vi "Process.vi"(8 "error in (no error)":errorcluster, 11 "SMO.UI.Example":refnum<class "SMO.UI.Example.lvclass">) -> (0 "error out":errorcluster, 3 "SMO.UI.Example out":refnum<class "SMO.UI.Example.lvclass">)   [LabVIEW 2013, in "SMO.UI.Example.lvclass"]
uses:
  SMO.UI.Example.lvclass
  src/SMO/Typedefs/Parent Call--Enum.ctl
  SMO.UI.Example.lvclass/SMO.UI.Example.ctl
  src/SMO.UI/SMO.UI.lvclass
  <vilib>/Utility/miscctls.llb/LVPointTypeDef.ctl
  SMO.Example/SMO.Example.lvclass
  src/SMO/SMO.lvclass
panel:
  in  "------------ User Events -------":bool=TRUE
  out "Waveform Chart":cluster{"Flow 2":dbl, "Flow 1":dbl}(graph)
  out "Sensor 1 (LPM)":u8
  out "Sensor 2 (LPM)":u8
  in  "Valve":bool
  in  "Pump":bool
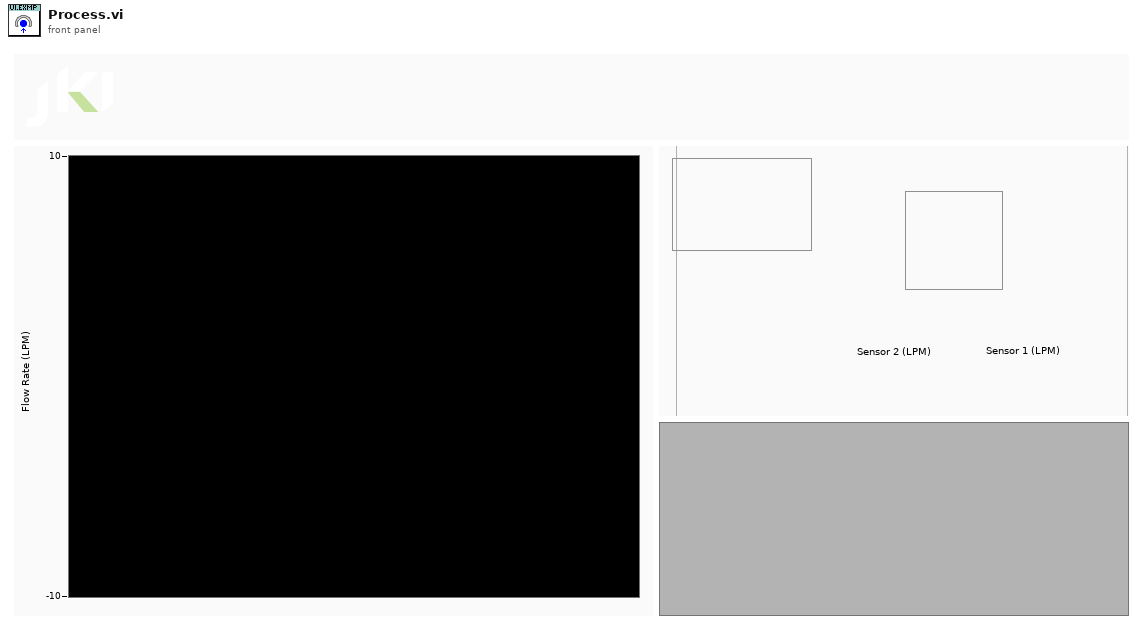
[diagram p1: front panel]
types:
  T1 = typedef "SMO.lvclass/Parent Call--Enum.ctl" = enum16{"Allows parent to run", "Does not request parent to run"}
  T2 = enum32{"invalid app kind", "Development System", "Run Time System", "Student Edition", "Embedded LabVIEW", "Evaluation", "Custom"}
  T3 = typedef "LVPointTypeDef.ctl" = cluster{"Horizontal":i16, "Vertical":i16}
  T4 = enum32{"Invalid", "Standard", "Closed", "Hidden", "Minimized", "Maximized"}
  T5 = typedef "SMO.UI.Example.lvclass/Dependencies--Cluster.ctl" = cluster{"SMO.Example":refnum<class "SMO.Example.lvclass">}
  T6 = cluster{"Core":cluster{"Current VI Reference":refnum<vi>, "Close Panel on Exit?":bool, "error":errorcluster}, "Self Ref":refnum<class "SMO.UI.Example.lvclass">, "Dependencies":T5, "Flow 1":dbl, "Flow 2":dbl, "Pump State":bool}
  T7 = cluster{"Current VI Reference":refnum<vi>, "Close Panel on Exit?":bool, "error":errorcluster}
  T8 = typedef "SMO.lvclass/Protected Events.ctl" = cluster{"StopProcesses":refnum<user-event>, "AbortProcesses":refnum<user-event>, "Config Changed":refnum<user-event>, "Dependency":refnum<user-event>}
  T9 = cluster{"Event Registration Refnum":refnum<event-registration>, "SMO.Example Public Events":refnum<event-registration>}
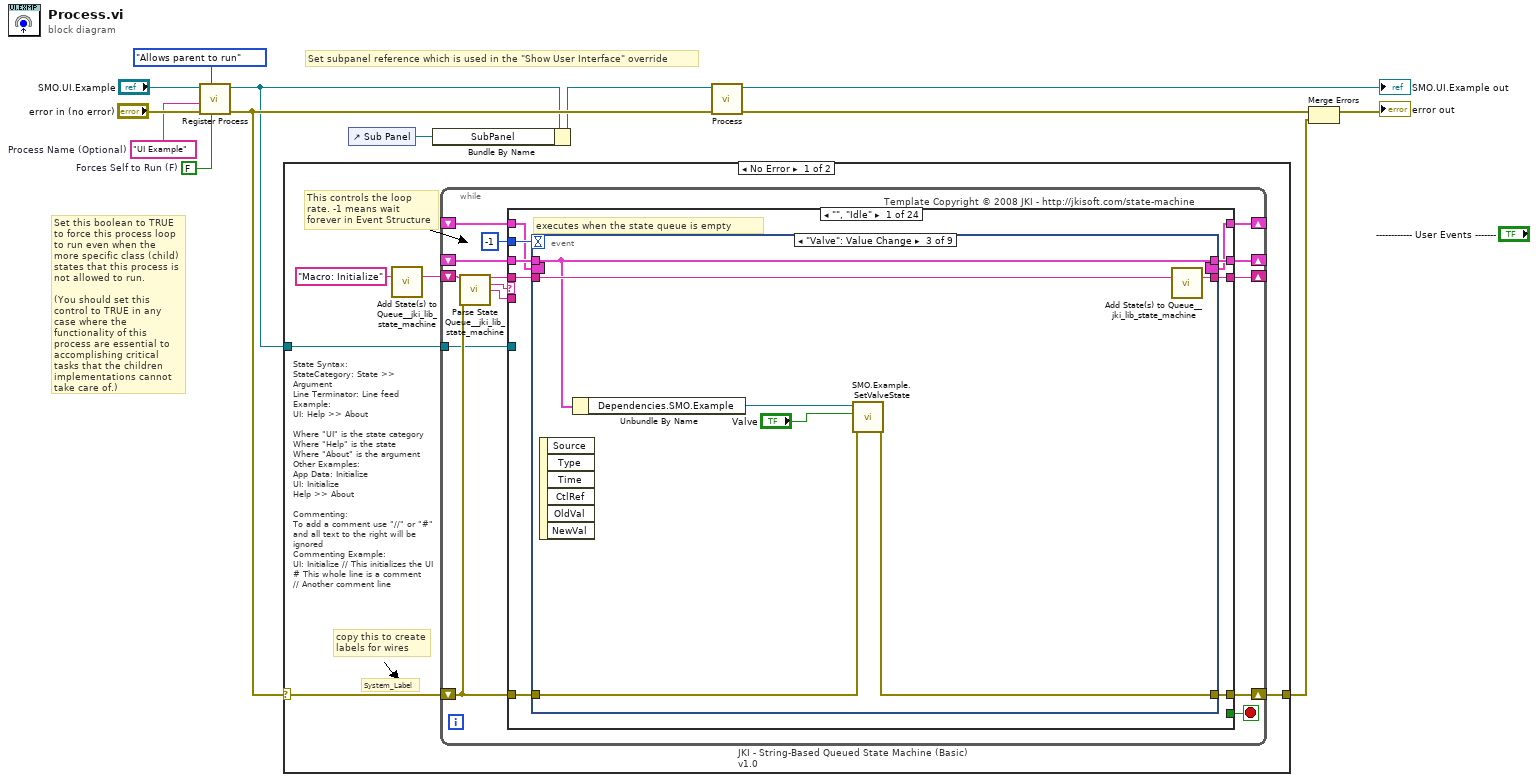
[diagram p0: block diagram]
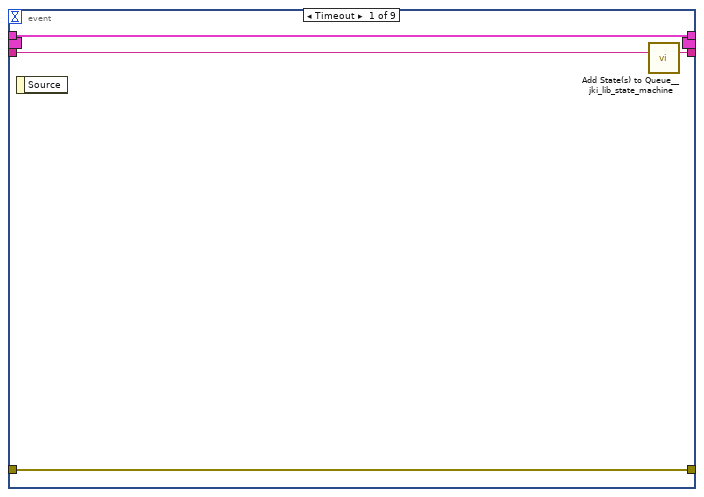
[diagram p2: hidden frame]
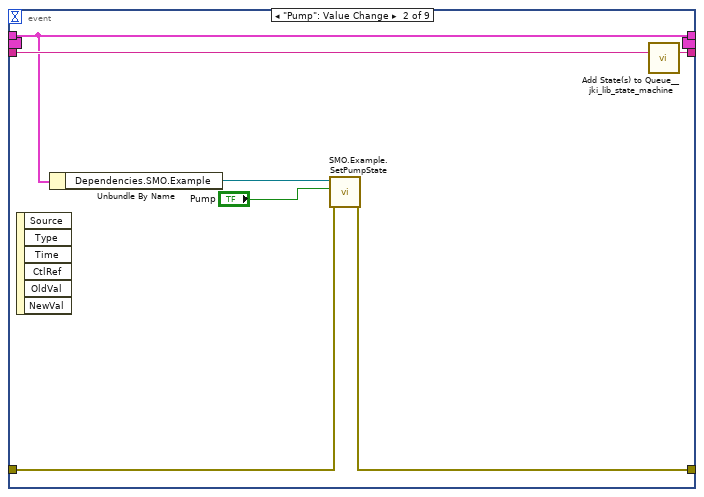
[diagram p3: hidden frame]
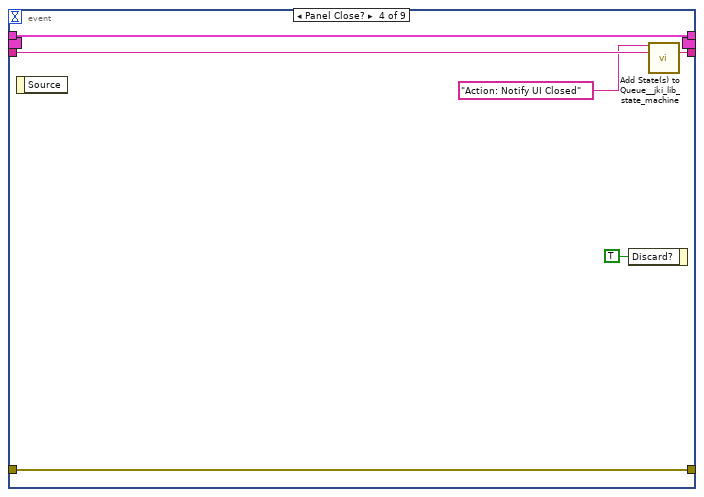
[diagram p4: hidden frame]
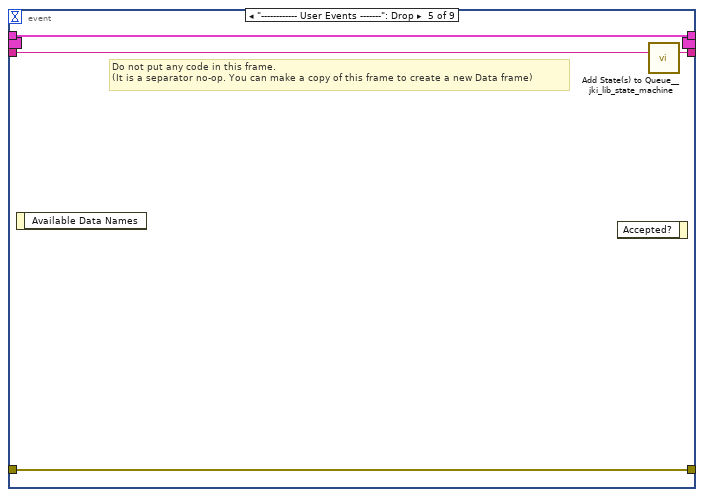
[diagram p5: hidden frame]
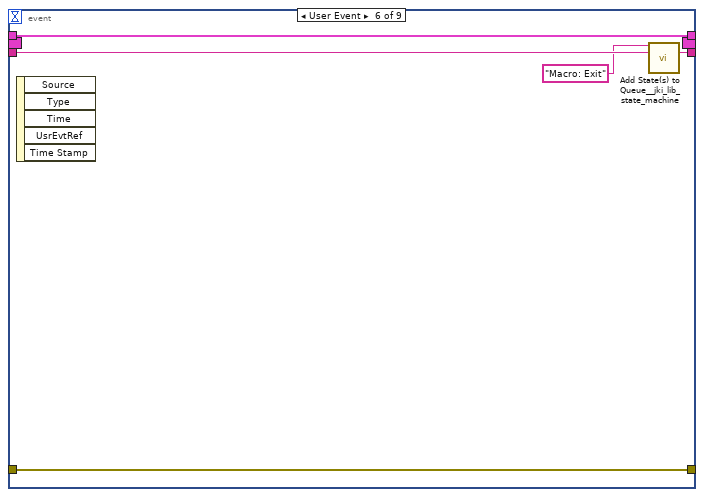
[diagram p6: hidden frame]
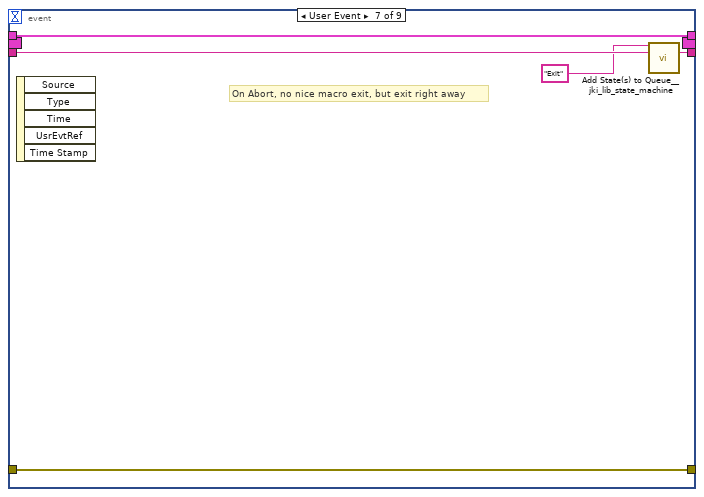
[diagram p7: hidden frame]
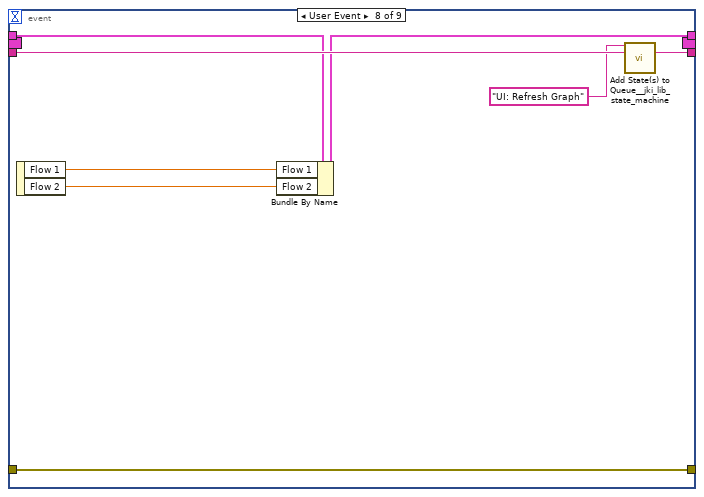
[diagram p8: hidden frame]
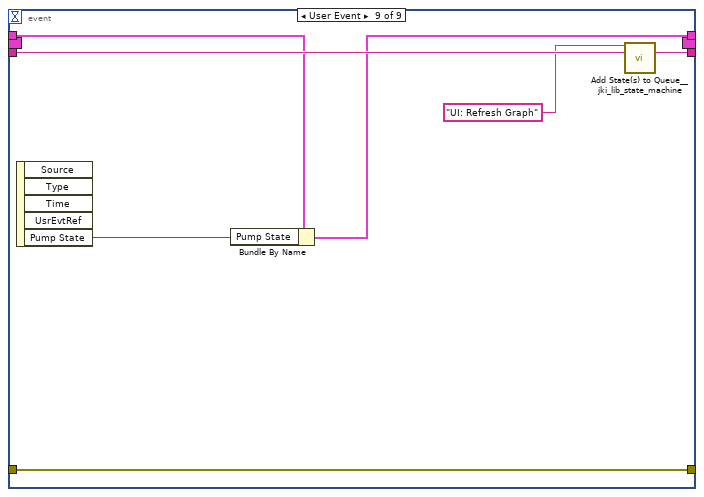
[diagram p9: hidden frame]
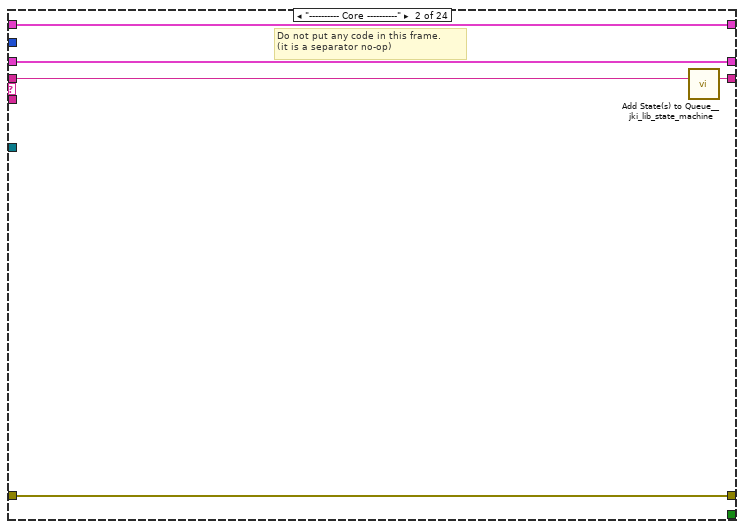
[diagram p10: hidden frame]
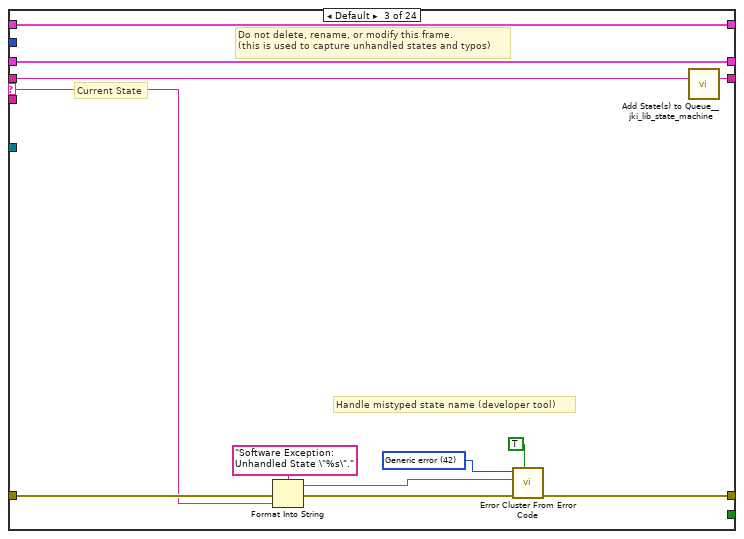
[diagram p11: hidden frame]
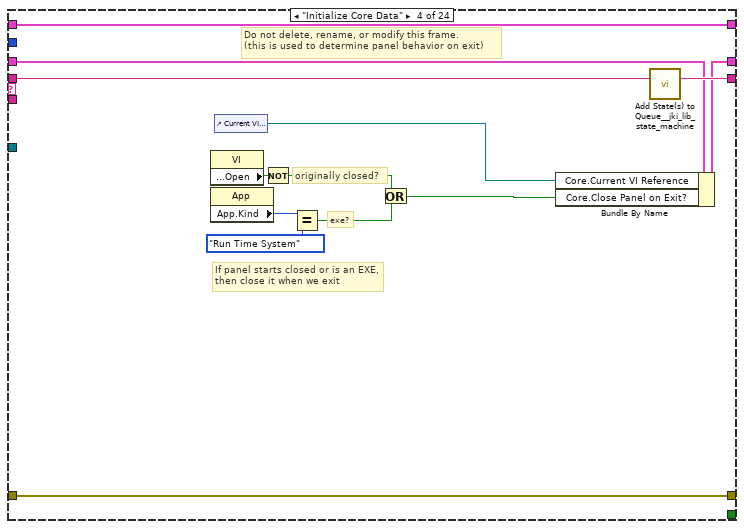
[diagram p12: hidden frame]
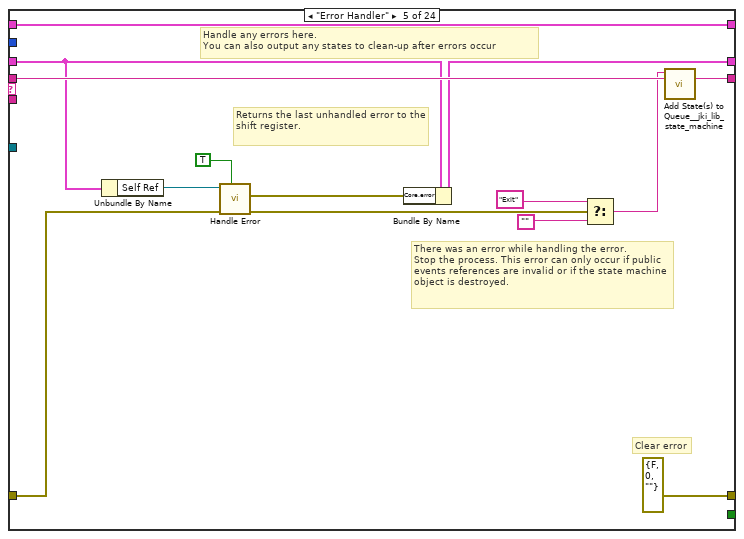
[diagram p13: hidden frame]
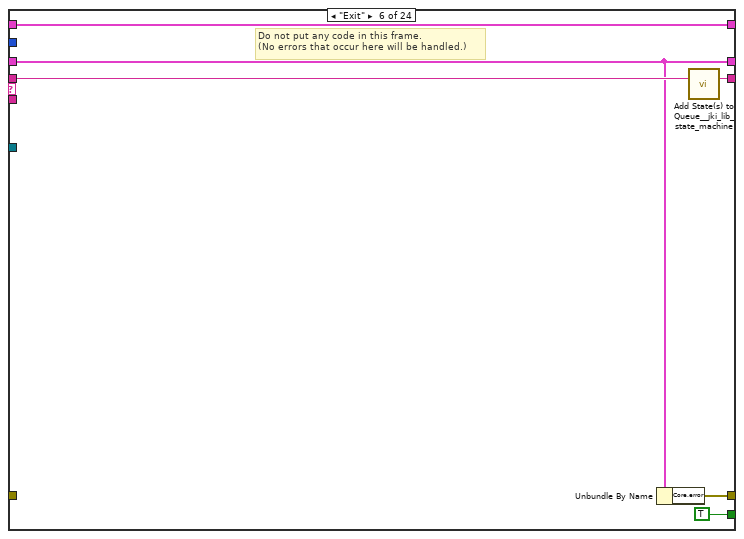
[diagram p14: hidden frame]
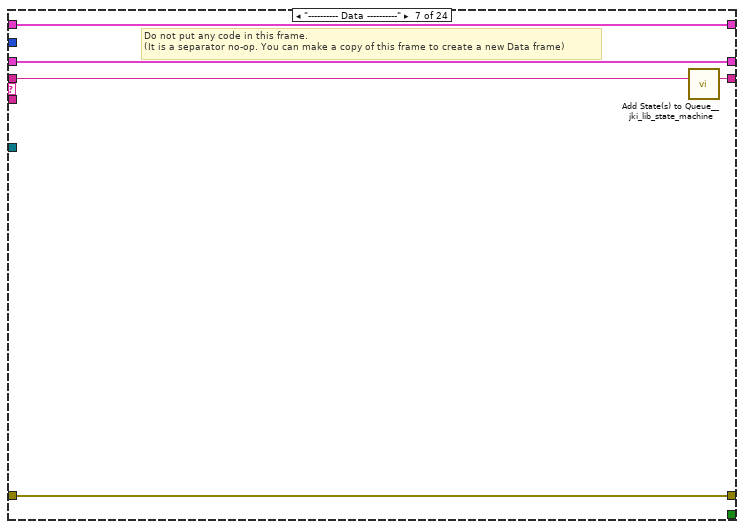
[diagram p15: hidden frame]
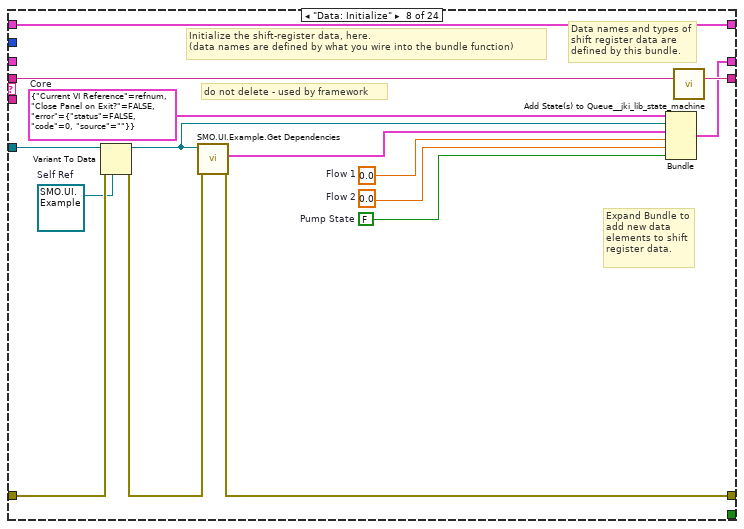
[diagram p16: hidden frame]
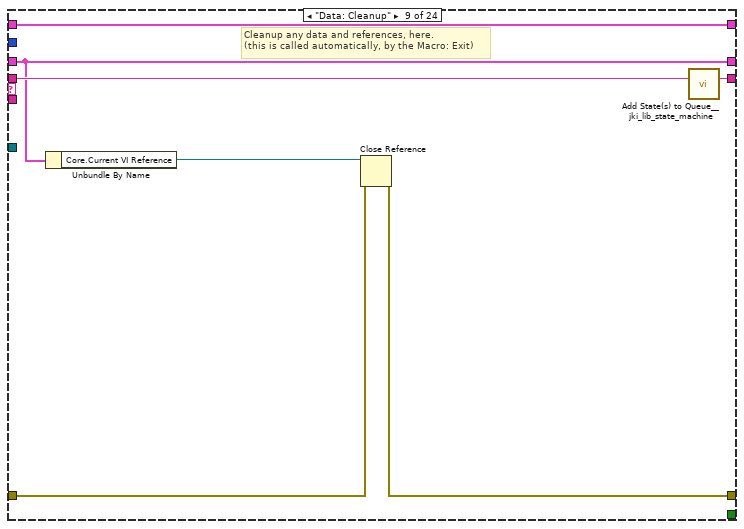
[diagram p17: hidden frame]
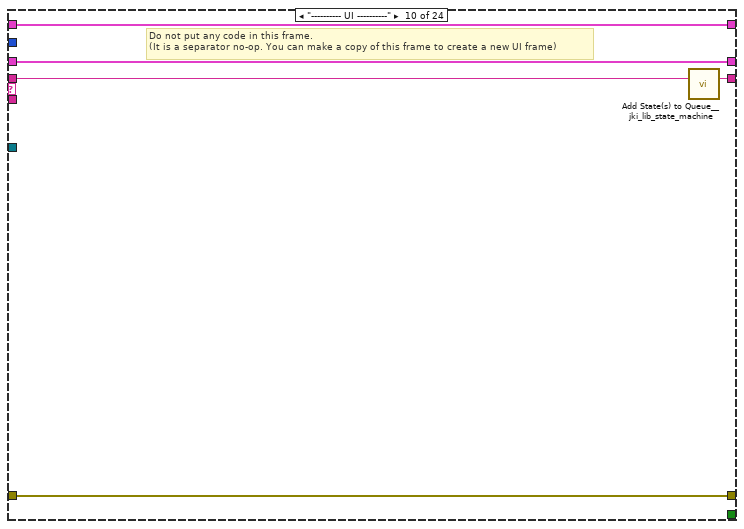
[diagram p18: hidden frame]
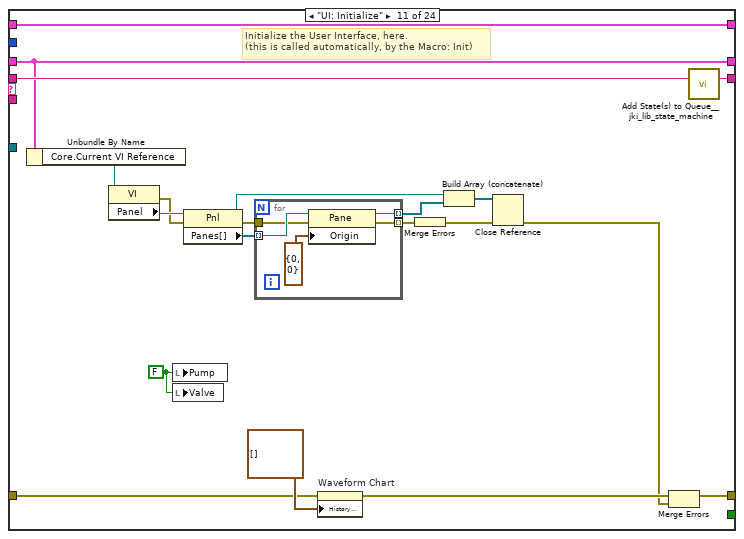
[diagram p19: hidden frame]
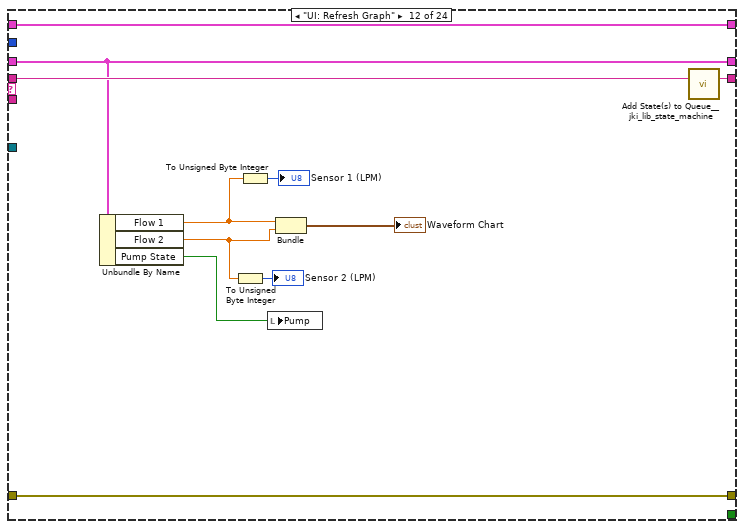
[diagram p20: hidden frame]
diagram:
  w1 = FALSE  # Forces Self to Run (F)
  w6 = "UI Example"  # Process Name (Optional)
  # "Set this boolean to TRUE to force this process loop to run even when the more specific class (child) states that this process is not allowed to run.\n\n(You should set this control to TRUE in any case where the functionality of this process are essential to accomplishing critical tasks that the children implementations cannot take care of.)"
  # "Set subpanel reference which is used in the \"Show User Interface\" override"
  n1 = call "Register Process.vi"("Forces Self to Run (F)"=w1, "Parent Call"=Parent_Call--Enum."Allows parent to run", "error in (no error)"="error in (no error)", "Process Name (optional)"=w6, "SMO"="SMO.UI.Example") -> ("error out"=w13:errorcluster, "SMO out"=w4:refnum<class "SMO.UI.Example.lvclass">)  [unwired: 5 in]
  n2 = case shown="No Error" w13 {
    selector: w13 -> [w15 w345]
    tunnel: w4 -> [w16 _]
    tunnel: [w14 w345] -> w11
    frame No Error {
      # "State Syntax:\nStateCategory: State >> Argument\nLine Terminator: Line feed\nExample:\nUI: Help >> About\n\nWhere \"UI\" is the state category\nWhere \"Help\" is the state\nWhere \"About\" is the argument\nOther Examples:\nApp Data: Initialize\nUI: Initialize\nHelp >> About\n\nCommenting:\nTo add a comment use \"//\" or \"#\" and all text to the right will be ignored\nCommenting Example:\nUI: Initialize // This initializes the UI\n# This whole line is a comment\n// Another comment line"
      # "copy this to create labels for wires"
      # "This controls the loop rate. -1 means wait forever in Event Structure"
      # "System_Label"
      n3 = call <vilib>:"Add State(s) to Queue__jki_lib_state_machine.vi"("State(s) in (\"\")"="Macro: Initialize") -> ("States Out"=w18:string)  [unwired: 14 in]
      n4 = while "JKI - String-Based Queued State Machine (Basic) v1.0" {
        shift-right: [w25] -> _
        shift-left: _ -> [w24]
        shift-right: [w28] -> w14
        shift-left: w15 -> [w22]
        shift-right: [w27] -> _
        shift-left: w18 -> [w29]
        tunnel: w16 -> [w21]
        shift-right: [w20] -> _
        shift-left: _ -> [w19]
        stop <- w26 stop-if-true
        # "Template Copyright © 2008 JKI - http://jkisoft.com/state-machine"
        n5 = call <vilib>:"Parse State Queue__jki_lib_state_machine.vi"("State Queue"=w29, "Error In (no error)"=w22) -> ("Remaining States"=w31:string, "Current State"=w32:string, "Arguments"=w30:string)  [unwired: 11 in]
        n6 = case shown="\"\", \"Idle\"" w32 {
          selector: w32 -> [_ _ w101 _ _ _ _ _ _ _ _ _ _ _ _ _ _ _ _ _ _ _ _ _]
          tunnel: w31 -> [w41 w99 w105 w124 w138 w144 w149 w164 w171 w176 w196 w212 w219 w235 w267 w276 w290 w295 w306 w311 w326 w332 w337 w344]
          tunnel: w30 -> [_ _ _ _ _ _ _ _ _ _ _ _ w213 w231 _ _ _ _ _ _ _ _ _ _]
          tunnel: w24 -> [w39 w96 w103 w115 w127 w140 w146 _ w166 w173 w191 w204 w217 w233 w264 w272 w281 w292 w303 w308 w324 w330 w334 w340]
          tunnel: [w38 w97 w107 w121 errorcluster {"status"=FALSE, "code"=0, "source"=""} ("error out") w139 w147 w153 w167 w174 w182 w203 w214 w228 w265 w274 w288 w293 w297 w309 w316 w328 w335 w338] -> w28
          tunnel: w22 -> [w37 w97 w106 w121 w129 _ w147 w161 w168 w174 w185 w203 w215 w229 w265 w274 w288 w293 w298 w309 w317 w328 w335 w339]
          tunnel: [w40 w98 w104 w123 w137 w143 w148 w163 w170 w175 w195 w211 w218 w234 w266 w275 w289 w294 w305 w310 w325 w331 w336 w343] -> w27
          tunnel: [_ _ _ _ _ TRUE _ _ _ _ _ _ _ _ _ _ _ _ _ _ _ _ _ _] -> w26
          tunnel: [w36 w96 w103 w122 w126 w140 w146 w162 w166 w173 w191 w204 w217 w233 w264 w272 w281 w292 w303 w308 w324 w330 w334 w340] -> w25
          tunnel: -1 ("Timeout") -> [w35 _ _ _ _ _ _ _ _ _ _ _ _ _ _ _ _ _ _ _ _ _ _ _]
          tunnel: w21 -> [_ _ _ _ _ _ _ w160 _ _ _ _ _ _ _ _ _ _ _ _ _ _ _ _]
          tunnel: [w33 w95 w100 w112 w135 w141 w145 w159 w165 w172 w192 w210 w216 w232 w263 w273 w282 w291 w304 w307 w319 w329 w333 w342] -> w20
          tunnel: w19 -> [w34 w95 w100 w112 w135 w141 w145 w159 w165 w172 w192 w210 w216 w232 w263 w273 w282 w291 w304 w307 _ w329 w333 w342]
          frame "", "Idle" {
            # "executes when the state queue is empty"
            n7 = event shown="[2] \"Valve\": Value Change" {
              selector: w34 -> [_ _ _ _ _ _ _ _ _]
              dyn-events: [_ _ _ _ _ _ _ _ _] -> w33
              timeout: w35 -> [_ _ _ _ _ _ _ _ _]
              tunnel: w41 -> [w45 w52 w59 w65 w69 w74 w79 w87 w94]
              tunnel: [w44 w51 w58 w64 w68 w73 w78 w86 w93] -> w40
              tunnel: w39 -> [w42 w50 w57 w63 w66 w71 w76 w83 w90]
              tunnel: [w43 w46 w54 w61 w67 w72 w77 w85 w92] -> w38
              tunnel: w37 -> [w43 w47 w55 w61 w67 w72 w77 w85 w92]
              tunnel: [w42 w50 w57 w63 w66 w71 w76 w84 w89] -> w36
              event Timeout {
                n8 = event-data() -> ()  [unwired: 1 in, 1 out]
                n9 = call <vilib>:"Add State(s) to Queue__jki_lib_state_machine.vi"("State(s) in (\"\")"=w45) -> ("States Out"=w44:string)  [unwired: 14 in]
              }
              event "Pump": Value Change {
                n10 = event-data() -> ()  [unwired: 1 in, 6 out]
                n11 = Unbundle By Name(w50) -> ("Dependencies.SMO.Example"=w49:refnum<class "SMO.Example.lvclass">)
                n12 = call "SMO.Example.SetPumpState.vi"("error in (no error)"=w47, "Pump State"="Pump", "SMO.Example"=w49) -> ("error out"=w46:errorcluster)  [unwired: 7 in, 1 out]
                n13 = call <vilib>:"Add State(s) to Queue__jki_lib_state_machine.vi"("State(s) in (\"\")"=w52) -> ("States Out"=w51:string)  [unwired: 14 in]
              }
              event "Valve": Value Change {
                n14 = event-data() -> ()  [unwired: 1 in, 6 out]
                n15 = Unbundle By Name(w57) -> ("Dependencies.SMO.Example"=w56:refnum<class "SMO.Example.lvclass">)
                n16 = call "SMO.Example.SetValveState.vi"("error in (no error)"=w55, "Valve State"="Valve", "SMO.Example"=w56) -> ("error out"=w54:errorcluster)  [unwired: 7 in, 1 out]
                n17 = call <vilib>:"Add State(s) to Queue__jki_lib_state_machine.vi"("State(s) in (\"\")"=w59) -> ("States Out"=w58:string)  [unwired: 14 in]
              }
              event Panel Close? {
                n18 = event-data() -> ()  [unwired: 1 in, 1 out]
                n19 = event-data("Discard?"=TRUE) -> ()  [unwired: 1 in, 1 out]
                n20 = call <vilib>:"Add State(s) to Queue__jki_lib_state_machine.vi"("State(s) in Front (\"\")"="Action: Notify UI Closed" ("State(s) in Front (\"\")"), "State(s) in (\"\")"=w65) -> ("States Out"=w64:string)  [unwired: 13 in]
              }
              event "------------ User Events -------": Drop {
                # "Do not put any code in this frame.\n(It is a separator no-op. You can make a copy of this frame to create a new Data frame)"
                n21 = event-data() -> ()  [unwired: 1 in, 1 out]
                n22 = event-data() -> ()  [unwired: 2 in, 1 out]
                n23 = call <vilib>:"Add State(s) to Queue__jki_lib_state_machine.vi"("State(s) in (\"\")"=w69) -> ("States Out"=w68:string)  [unwired: 14 in]
              }
              event User Event {
                n24 = event-data() -> ()  [unwired: 1 in, 5 out]
                n25 = call <vilib>:"Add State(s) to Queue__jki_lib_state_machine.vi"("State(s) in Front (\"\")"="Macro: Exit", "State(s) in (\"\")"=w74) -> ("States Out"=w73:string)  [unwired: 13 in]
              }
              event User Event {
                # "On Abort, no nice macro exit, but exit right away"
                n26 = event-data() -> ()  [unwired: 1 in, 5 out]
                n27 = call <vilib>:"Add State(s) to Queue__jki_lib_state_machine.vi"("State(s) in Front (\"\")"="Exit", "State(s) in (\"\")"=w79) -> ("States Out"=w78:string)  [unwired: 13 in]
              }
              event User Event {
                n28 = event-data() -> ("Flow 1"=w82:dbl, "Flow 2"=w81:dbl)  [unwired: 1 in]
                n29 = Bundle By Name(cluster=w83, "Flow 1"=w82, "Flow 2"=w81) -> (w84:T6)
                n30 = call <vilib>:"Add State(s) to Queue__jki_lib_state_machine.vi"("State(s) in Front (\"\")"="UI: Refresh Graph", "State(s) in (\"\")"=w87) -> ("States Out"=w86:string)  [unwired: 13 in]
              }
              event User Event {
                n31 = event-data() -> ("Pump State"=w91:bool)  [unwired: 1 in, 4 out]
                n32 = Bundle By Name(cluster=w90, "Pump State"=w91) -> (w89:T6)
                n33 = call <vilib>:"Add State(s) to Queue__jki_lib_state_machine.vi"("State(s) in Front (\"\")"="UI: Refresh Graph", "State(s) in (\"\")"=w94) -> ("States Out"=w93:string)  [unwired: 13 in]
              }
            }
          }
          frame "---------- Core ----------" {
            # "Do not put any code in this frame.\n(it is a separator no-op)"
            n34 = call <vilib>:"Add State(s) to Queue__jki_lib_state_machine.vi"("State(s) in (\"\")"=w99) -> ("States Out"=w98:string)  [unwired: 14 in]
          }
          frame Default {
            w110 = 42 items=["No error", "Argument error", "Memory is full", "Out of zone", "End of file", "File already open", "Generic file I/O error", "File not found", "File permission error", "Disk is full", "Duplicate path", "Too many files open", "System feature not enabled", "Resource file not found", "Cannot add resource", "Resource not found", "Image not found", "Image memory error", "Pen does not exist", "Config type invalid", "Config token not found", "Config parse error", "Config memory error", "Bad external code format", "Bad external code offset", "External code not present", "Null window", "Destroy window error", "Null menu", "Print aborted", "Bad print record", "Print driver error", "Windows error during printing", "Memory error during printing", "Print dialog error", "Generic print error", "Invalid device refnum", "Device not found", "Device parameter error", "Device unit error", "Cannot open device", "Device call aborted", "Generic error", "Cancelled by user", "Object ID too low", "Object ID too high", "Object not in heap", "Unknown heap", "Unknown object (invalid DefProc)", "Unknown object (DefProc not in table)", "Message out of range", "Invalid (null) method", "Unknown message", "Manager call not supported", "Bad address", "Network operation in progress", "Network operation timed out", "Connection is busy", "Network attribute not supported", "Network error", "Address in use", "System out of memory", "Connection aborted", "Connection refused", "Not connected", "Already connected", "Connection closed", "Initialization error (interapplication manager)", "Bad occurrence", "Wait on unbound occurrence handler", "Occurrence queue overflow", "Datalog type conflict", "Unused", "Unrecognized type (interapplication manager)", "Memory corrupt", "Failed to make temporary DLL", "Old CIN version", "Drag socket not found", "Failed to load drop-object", "Failed to register OLE object", "Failed to release OLE object", "Format specifier type mismatch", "Unknown format specifier", "Too few format specifiers", "Too many format specifiers", "Scan failed", "Newer CIN version", "Error converting to variant", "Runtime menu error", "Password tampered", "Variant attribute not found", "Incompatible variant data type", "Event data is not available", "Event Store is not present", "Occurrence is not found", "Event Queue is not created", "Event info is not available", "Refnum passed is NULL", "Error retrieving Class GUID", "Error retrieving CoClass GUID", "Error retrieving TypeLib GUID.", "Bad built application magic bytes.", "Specific driver is different from the specific driver associated with the Logical Name.", "There is no session opened to the class driver.", "Max Error", "MAX - Error with config objects", "MAX - Error loading configuration", "MAX - Group not supported"]
            # "Current State"
            # "Do not delete, rename, or modify this frame.\n(this is used to capture unhandled states and typos)"
            # "Handle mistyped state name (developer tool)"
            n35 = Format Into String(format string="Software Exception: Unhandled State \"%s\"." ("message"), error in=w106, w101) -> (resulting string=w109:string, error out=w108:errorcluster)  [unwired: 1 in]
            n36 = call <vilib>:"Error Cluster From Error Code.vi"("show call chain? (False)"=TRUE, "error in (no error)"=w108, "error message (\"\")"=w109, "error code (0)"=w110) -> ("error out"=w107:errorcluster)  [unwired: 5 in]
            n37 = call <vilib>:"Add State(s) to Queue__jki_lib_state_machine.vi"("State(s) in (\"\")"=w105) -> ("States Out"=w104:string)  [unwired: 14 in]
          }
          frame "Initialize Core Data" {
            # "Do not delete, rename, or modify this frame.\n(this is used to determine panel behavior on exit)"
            # "originally closed?"
            # "exe?"
            # "If panel starts closed or is an EXE, then close it when we exit"
            n38 = property class="VI"() -> ("Front Panel.Open"=w120:bool)  [unwired: 2 in, 2 out]
            n39 = property class="App"() -> ("App.Kind"=w119:T2)  [unwired: 2 in, 2 out]
            n40 = control-ref of="Current VI Reference"() -> (w113:refnum<vi>)
            n41 = Not(x=w120) -> (.not. x?=w117:bool)
            n42 = Equal?(x=w119, y=T2."Run Time System" ("Application:Kind")) -> (x = y?=w116:bool)
            n43 = Or(x=w117, y=w116) -> (x .or. y?=w114:bool)
            n44 = Bundle By Name(cluster=w115, "Core.Current VI Reference"=w113, "Core.Close Panel on Exit?"=w114) -> (w122:T6)
            n45 = call <vilib>:"Add State(s) to Queue__jki_lib_state_machine.vi"("State(s) in (\"\")"=w124) -> ("States Out"=w123:string)  [unwired: 14 in]
          }
          frame "Error Handler" {
            # "Returns the last unhandled error to the shift register."
            # "There was an error while handling the error.\nStop the process. This error can only occur if public events references are invalid or if the state machine object is destroyed."
            # "Handle any errors here.\nYou can also output any states to clean-up after errors occur"
            # "Clear error"
            n46 = Unbundle By Name(w127) -> ("Self Ref"=w134:refnum<class "SMO.UI.Example.lvclass">)
            n47 = call-dynamic "Handle Error.vi"("Stop on Unhandled Error (T)"=TRUE, "error in"=w129, "SMO"=w134) -> ("handling error"=w132:errorcluster, "Unhandled error"=w133:errorcluster)  [unwired: 6 in, 1 out]
            n48 = Bundle By Name(cluster=w127, "Core.error"=w133) -> (w126:T6)
            n49 = Select(t="Exit", s=w132, f="") -> (s? t:f=w128:string)
            n50 = call <vilib>:"Add State(s) to Queue__jki_lib_state_machine.vi"("State(s) in Front (\"\")"=w128, "State(s) in (\"\")"=w138) -> ("States Out"=w137:string)  [unwired: 13 in]
          }
          frame "Exit" {
            # "Do not put any code in this frame.\n(No errors that occur here will be handled.)"
            n51 = Unbundle By Name(w140) -> ("Core.error"=w139:errorcluster)
            n52 = call <vilib>:"Add State(s) to Queue__jki_lib_state_machine.vi"("State(s) in (\"\")"=w144) -> ("States Out"=w143:string)  [unwired: 14 in]
          }
          frame "---------- Data ----------" {
            # "Do not put any code in this frame.\n(It is a separator no-op. You can make a copy of this frame to create a new Data frame)"
            n53 = call <vilib>:"Add State(s) to Queue__jki_lib_state_machine.vi"("State(s) in (\"\")"=w149) -> ("States Out"=w148:string)  [unwired: 14 in]
          }
          frame "Data: Initialize" {
            w150 = FALSE  # Pump State
            w152 = 0.0  # Flow 1
            w151 = 0.0  # Flow 2
            w157 = refnum<class "SMO.UI.Example.lvclass"> refnum  # Self Ref
            w158 = T7 {"Current VI Reference"=refnum, "Close Panel on Exit?"=FALSE, "error"={"status"=FALSE, "code"=0, "source"=""}}  # Core
            # "do not delete - used by framework"
            # "Expand Bundle to add new data elements to shift register data."
            # "Data names and types of shift register data are defined by this bundle."
            # "Initialize the shift-register data, here.\n(data names are defined by what you wire into the bundle function)"
            n54 = Variant To Data(error in=w161, type=w157, Variant=w160) -> (data=w155:refnum<class "SMO.UI.Example.lvclass">, error out=w154:errorcluster)
            n55 = call "SMO.UI.Example.Get Dependencies.vi"("error in (no error)"=w154, "SMO UI.Template in"=w155) -> ("error out"=w153:errorcluster, "Dependencies"=w156:T5)  [unwired: 7 in, 1 out]
            n56 = Bundle("Core"=w158, "Self Ref"=w155, "Dependencies"=w156, "Flow 1"=w152, "Flow 2"=w151, "Pump State"=w150) -> (w162:T6)  [unwired: 1 in]
            n57 = call <vilib>:"Add State(s) to Queue__jki_lib_state_machine.vi"("State(s) in (\"\")"=w164) -> ("States Out"=w163:string)  [unwired: 14 in]
          }
          frame "Data: Cleanup" {
            # "Cleanup any data and references, here.\n(this is called automatically, by the Macro: Exit)"
            n58 = Unbundle By Name(w166) -> ("Core.Current VI Reference"=w169:refnum<vi>)
            n59 = Close Reference(reference=w169, error in (no error)=w168) -> (error out=w167:errorcluster)
            n60 = call <vilib>:"Add State(s) to Queue__jki_lib_state_machine.vi"("State(s) in (\"\")"=w171) -> ("States Out"=w170:string)  [unwired: 14 in]
          }
          frame "---------- UI ----------" {
            # "Do not put any code in this frame.\n(It is a separator no-op. You can make a copy of this frame to create a new UI frame)"
            n61 = call <vilib>:"Add State(s) to Queue__jki_lib_state_machine.vi"("State(s) in (\"\")"=w176) -> ("States Out"=w175:string)  [unwired: 14 in]
          }
          frame "UI: Initialize" {
            w194 = FALSE ("Pump")
            # "Initialize the User Interface, here.\n(this is called automatically, by the Macro: Init)"
            n62 = Unbundle By Name(w191) -> ("Core.Current VI Reference"=w190:refnum<vi>)
            n63 = property class="VI"(reference=w190) -> (error out=w187:errorcluster, "Panel"=w189:refnum<vi>)  [unwired: 1 in, 1 out]
            n64 = local write "Pump"(w194) -> ()
            n65 = local write "Valve"(w194) -> ()
            n66 = property class="Pnl"(reference=w189, error in=w187) -> (reference out=w181:refnum<vi>, error out=w186:errorcluster, "Panes[]"=w188:refnum<vi>[])
            n67 = for {
              tunnel: w188 -> [w201] mode=indexing
              tunnel: w186 -> [w199]
              tunnel: [w198] -> w184 mode=indexing
              tunnel: [w197] -> w180 mode=indexing
              n68 = property class="Pane"(reference=w201, error in=w199, "Origin"=T3 {"Horizontal"=0, "Vertical"=0}) -> (reference out=w197:refnum<vi>, error out=w198:errorcluster)
            }
            n69 = property on="Waveform Chart" class="WFChart (strict)"(error in=w185, "History Data"=cluster{"Flow 2":dbl, "Flow 1":dbl}[] []) -> (error out=w183:errorcluster)  [unwired: 1 in, 1 out]
            n70 = Merge Errors(w184) -> (w179:errorcluster)
            n71 = Build Array (concatenate)(w181, w180) -> (w177:refnum<vi>[])
            n72 = Close Reference(reference=w177, error in (no error)=w179) -> (error out=w178:errorcluster)
            n73 = Merge Errors(w183, w178) -> (w182:errorcluster)
            n74 = call <vilib>:"Add State(s) to Queue__jki_lib_state_machine.vi"("State(s) in (\"\")"=w196) -> ("States Out"=w195:string)  [unwired: 14 in]
          }
          frame "UI: Refresh Graph" {
            n75 = Unbundle By Name(w204) -> ("Flow 1"=w207:dbl, "Flow 2"=w208:dbl, "Pump State"=w202:bool)
            n76 = To Unsigned Byte Integer(number=w208) -> (unsigned 8bit integer=→"Sensor 2 (LPM)":u8)
            n77 = To Unsigned Byte Integer(number=w207) -> (unsigned 8bit integer=→"Sensor 1 (LPM)":u8)
            n78 = local write "Pump"(w202) -> ()
            n79 = Bundle("Flow 1"=w207, "Flow 2"=w208) -> (→"Waveform Chart":cluster{"Flow 1":dbl, "Flow 2":dbl})  [unwired: 1 in]
            n80 = call <vilib>:"Add State(s) to Queue__jki_lib_state_machine.vi"("State(s) in (\"\")"=w212) -> ("States Out"=w211:string)  [unwired: 14 in]
          }
          frame "UI: Cursor Set" {
            # "Argument"
            # "Initialize the User Interface, here.\n(this is called automatically, by the Macro: Init)"
            n81 = disable-structure shown="Default" {
              disable-tunnel: w215 -> [w220 w223]
              disable-tunnel: [w220 w222] -> w214
              disable-tunnel: w213 -> [_ w221]
              frame condition #0 {
              }
              frame condition #1 (active) {
                n82 = case shown="\"Idle\", Default" w221 {
                  tunnel: w223 -> [w225 w227]
                  tunnel: [w224 w226] -> w222
                  frame "Idle", Default {
                    n83 = call <vilib>:"Unset Busy.vi"("error in (no error)"=w225) -> ("error out"=w224:errorcluster)  [unwired: 10 in]
                  }
                  frame "Busy" {
                    n84 = call <vilib>:"Set Busy.vi"("error in (no error)"=w227) -> ("error out"=w226:errorcluster)  [unwired: 9 in, 1 out]
                  }
                }
              }
            }
            n85 = call <vilib>:"Add State(s) to Queue__jki_lib_state_machine.vi"("State(s) in (\"\")"=w219) -> ("States Out"=w218:string)  [unwired: 14 in]
          }
          frame "UI: Front Panel State" {
            # "Argument"
            # "Set Front Panel Open or Closed\n(Usage: \"UI: Front Panel State >> Open|Close\")"
            n86 = Unbundle By Name(w233) -> ("Core.Current VI Reference"=w230:refnum<vi>)
            n87 = disable-structure shown="Default" {
              disable-tunnel: w229 -> [w239 w262]
              disable-tunnel: [w238 w262] -> w228
              disable-tunnel: w230 -> [w237 _]
              disable-tunnel: w231 -> [w236 _]
              frame condition #0 (active) {
                n88 = case shown="\"Open\", Default" w236 {
                  tunnel: w239 -> [w243 w256]
                  tunnel: [w245 w257] -> w238
                  tunnel: w237 -> [w244 w254]
                  frame "Open", Default {
                    # "Open FP if not open or invalid"
                    n89 = property class="VI"(reference=w244, error in=w243) -> (reference out=w241:refnum<vi>, error out=w242:errorcluster, "FP.State"=w240:T4)
                    n90 = case shown="Default" w240 {
                      tunnel: [w248 w251] -> w245
                      tunnel: w242 -> [w247 w251]
                      tunnel: w241 -> [w246 _]
                      frame Default {
                        n91 = invoke class="VI" method="FP.Open"(reference=w246, error in=w247, "Activate"=TRUE, "State"=T4."Standard") -> (error out=w248:errorcluster)  [unwired: 1 in, 4 out]
                      }
                      frame "Invalid", "Standard" {
                      }
                    }
                  }
                  frame "Close" {
                    # "Close FP is not Closed or Invalid"
                    n92 = property class="VI"(reference=w254, error in=w256) -> (reference out=w253:refnum<vi>, error out=w255:errorcluster, "FP.State"=w252:T4)
                    n93 = case shown="Default" w252 {
                      tunnel: [w258 w261] -> w257
                      tunnel: w255 -> [w258 w260]
                      tunnel: w253 -> [_ w259]
                      frame "Invalid", "Closed" {
                      }
                      frame Default {
                        n94 = invoke class="VI" method="FP.Close"(reference=w259, error in=w260) -> (error out=w261:errorcluster)  [unwired: 1 in, 2 out]
                      }
                    }
                  }
                }
              }
              frame condition #1 {
              }
            }
            n95 = call <vilib>:"Add State(s) to Queue__jki_lib_state_machine.vi"("State(s) in (\"\")"=w235) -> ("States Out"=w234:string)  [unwired: 14 in]
          }
          frame "---------- Macro ----------" {
            # "Do not put any code in this frame.\n(It is a separator no-op. You can make a copy of this frame to create a new Macro frame)"
            n96 = call <vilib>:"Add State(s) to Queue__jki_lib_state_machine.vi"("State(s) in (\"\")"=w267) -> ("States Out"=w266:string)  [unwired: 14 in]
          }
          frame "Macro: Initialize" {
            w270 = "UI: Initialize\n//UI: Front Panel State >> Open"  # UI: Initialize //UI: Front Panel State >> Open
            # "Initialization Macro\n(This is called once, when the VI starts)"
            n97 = call <vilib>:"Add State(s) to Queue__jki_lib_state_machine.vi"("State(s) in Front (\"\")"="Data: Initialize\nInitialize Core Data\nEvents: Register", "State(s) in (\"\")"="Process: Sync", "State(s) at Back (\"\")"=w270) -> ("States Out"=w269:string)  [unwired: 12 in]
            n98 = call <vilib>:"Add State(s) to Queue__jki_lib_state_machine.vi"("State(s) in Front (\"\")"=w269, "State(s) in (\"\")"=w276) -> ("States Out"=w275:string)  [unwired: 13 in]
          }
          frame "Macro: Exit" {
            # "Exit Macro\n(This is called once, when the VI exits)"
            n99 = Unbundle By Name(w281) -> ("Core.Close Panel on Exit?"=w287:bool)
            n100 = Select(t="//UI: Front Panel State >> Close", s=w287, f="") -> (s? t:f=w284:string)
            n101 = call <vilib>:"Add State(s) to Queue__jki_lib_state_machine.vi"("State(s) in Front (\"\")"="Data: Cleanup\nEvents: Unregister", "State(s) in (\"\")"="Process: Sync", "State(s) at Back (\"\")"="Exit") -> ("States Out"=w278:string)  [unwired: 12 in]
            n102 = call <vilib>:"Add State(s) to Queue__jki_lib_state_machine.vi"("State(s) in (\"\")"=w284, "State(s) at Back (\"\")"=w278) -> ("States Out"=w283:string)  [unwired: 13 in]
            n103 = call <vilib>:"Add State(s) to Queue__jki_lib_state_machine.vi"("State(s) in Front (\"\")"=w283, "State(s) in (\"\")"=w290) -> ("States Out"=w289:string)  [unwired: 13 in]
          }
          frame "---------- Process ----------" {
            # "Template Separator\n(You can make a copy of, or modify, this frame)"
            n104 = call <vilib>:"Add State(s) to Queue__jki_lib_state_machine.vi"("State(s) in (\"\")"=w295) -> ("States Out"=w294:string)  [unwired: 14 in]
          }
          frame "Process: Sync" {
            n105 = Unbundle By Name(w303) -> ("Self Ref"=w299:refnum<class "SMO.UI.Example.lvclass">)
            n106 = call "WaitOnProcessSync.vi"("error in (no error)"=w298, "SMO"=w299) -> ("error out"=w297:errorcluster, "Don't run?"=w302:bool)  [unwired: 7 in, 1 out]
            n107 = Select(t="Data: Cleanup\nEvents: Unregister\nExit", s=w302, f="") -> (s? t:f=w296:string)
            n108 = call <vilib>:"Add State(s) to Queue__jki_lib_state_machine.vi"("State(s) in Front (\"\")"=w296, "State(s) in (\"\")"=w306) -> ("States Out"=w305:string)  [unwired: 13 in]
          }
          frame "---------- Events ----------" {
            # "Template Separator\n(You can make a copy of, or modify, this frame)"
            n109 = call <vilib>:"Add State(s) to Queue__jki_lib_state_machine.vi"("State(s) in (\"\")"=w311) -> ("States Out"=w310:string)  [unwired: 14 in]
          }
          frame "Events: Register" {
            # "Clear error when dependency not created. (Demo only)"
            # "Dependency Public Events"
            # "Base Class Protected Events"
            n110 = Unbundle By Name(w324) -> ("Self Ref"=w318:refnum<class "SMO.UI.Example.lvclass">)
            n111 = Unbundle By Name(w324) -> ("Dependencies.SMO.Example"=w322:refnum<class "SMO.Example.lvclass">)
            n112 = call "SMO.Example.GetPublicEventsRegistration.vi"("SMO.Example"=w322) -> ("error out"=w313:errorcluster, "SMO.Example Public Events"=w321:refnum<event-registration>)  [unwired: 8 in, 1 out]
            n113 = call <vilib>:"Clear Errors.vi"("error in (no error)"=w313) -> ("error out"=w312:errorcluster)  [unwired: 6 in]
            n114 = call "GetProtectedEvents.vi"("SMO"=w318) -> ("error out"=w314:errorcluster, "SMO Protected Events"=w323:T8)  [unwired: 8 in, 1 out]
            n115 = register-events(w323) -> (reference out=w320:refnum<event-registration>, error out=w315:errorcluster)  [unwired: 2 in]
            n116 = Merge Errors(w315, w314, w312, w317) -> (w316:errorcluster)
            n117 = Bundle("Event Registration Refnum"=w320, "SMO.Example Public Events"=w321) -> (w319:T9)  [unwired: 1 in]
            n118 = call <vilib>:"Add State(s) to Queue__jki_lib_state_machine.vi"("State(s) in (\"\")"=w326) -> ("States Out"=w325:string)  [unwired: 14 in]
          }
          frame "Events: Unregister" {
            n119 = Unregister For Events(event registration refnum=w329, error in=w328) -> (error out=w327:errorcluster)
            n120 = call <vilib>:"Clear Errors.vi"("error in (no error)"=w327) -> ()  [unwired: 6 in, 1 out]
            n121 = call <vilib>:"Add State(s) to Queue__jki_lib_state_machine.vi"("State(s) in (\"\")"=w332) -> ("States Out"=w331:string)  [unwired: 14 in]
          }
          frame "---------Action---------" {
            # "Action Separator\n(You can make a copy of, or modify, this frame)"
            n122 = call <vilib>:"Add State(s) to Queue__jki_lib_state_machine.vi"("State(s) in (\"\")"=w337) -> ("States Out"=w336:string)  [unwired: 14 in]
          }
          frame "Action: Notify UI Closed" {
            # "Notify that the UI has closed"
            # "Action Separator\n(You can make a copy of, or modify, this frame)"
            n123 = Unbundle By Name(w340) -> ("Self Ref"=w341:refnum<class "SMO.UI.Example.lvclass">)
            n124 = call "Hide.vi"("error in (no error)"=w339, "SMO.UI"=w341) -> ("error out"=w338:errorcluster)  [unwired: 8 in, 1 out]
            n125 = call <vilib>:"Add State(s) to Queue__jki_lib_state_machine.vi"("State(s) in (\"\")"=w344) -> ("States Out"=w343:string)  [unwired: 14 in]
          }
        }
      }
    }
    frame Error {
    }
  }
  n126 = control-ref of="Sub Panel"() -> (w2:refnum<vi>)
  n127 = Bundle By Name(cluster=w4, "SubPanel"=w2) -> (w3:refnum<class "SMO.UI.Example.lvclass">)
  n128 = call-parent "Process.vi"("error in (no error)"=w13, "SMO.UI"=w3) -> ("error out"=w12:errorcluster, "SMO.UI out"=→"SMO.UI.Example out":refnum<class "SMO.UI.Example.lvclass">)  [unwired: 8 in]
  n129 = Merge Errors(w12, w11) -> (→"error out":errorcluster)
